vi "Write Elapsed (ms).vi"(8 "error in (no error)":errorcluster, 10 "Elapsed (ms)":i32, 11 "Wait On Boolean Step in":refnum<class "Wait On Boolean Step.lvclass">) -> (0 "error out":errorcluster, 3 "Wait On Boolean Step out":refnum<class "Wait On Boolean Step.lvclass">)   [LabVIEW 2015, in "Wait On Boolean Step.lvclass"]
uses:
  Wait On Boolean Step.lvclass
  Wait On Boolean Step.lvclass/Wait On Boolean Step.ctl
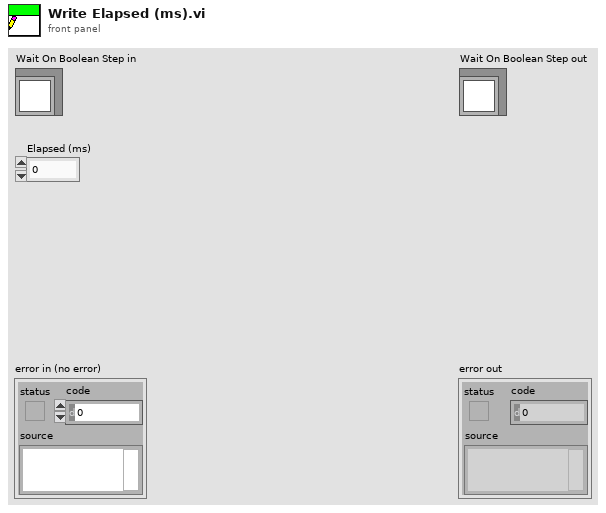
[diagram p1: front panel]
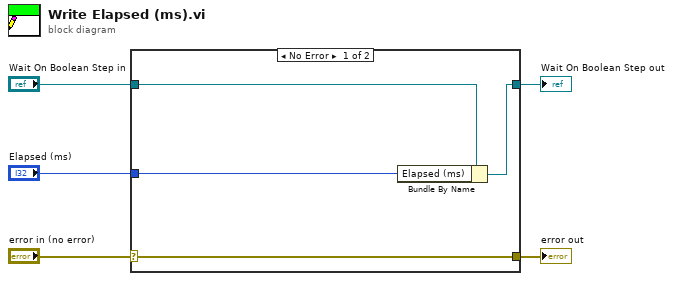
[diagram p0: block diagram]
diagram:
  n1 = case shown="No Error" "error in (no error)" {
    selector: "error in (no error)" -> [w9 w10]
    tunnel: [w9 w10] -> w4
    tunnel: [w7 w11] -> w2
    tunnel: "Wait On Boolean Step in" -> [w8 w11]
    tunnel: "Elapsed (ms)" -> [w6 _]
    frame No Error {
      n2 = Bundle By Name(cluster=w8, "Elapsed (ms)"=w6) -> (w7:refnum<class "Wait On Boolean Step.lvclass">)
    }
    frame Error {
    }
  }
  "error out" <- w4
  "Wait On Boolean Step out" <- w2
